vi "device name shot number from tcp udp.vi"(11 "ShotData UDP response":string) -> (1 "all data":string, 2 "shot number":string, 3 "Device name":string)   [LabVIEW 2013]
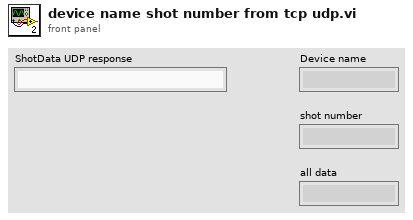
[diagram p1: front panel]
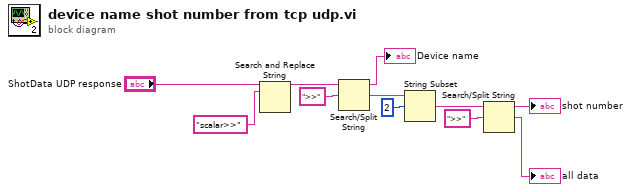
[diagram p0: block diagram]
diagram:
  n1 = Search and Replace String(input string="ShotData UDP response", search string="scalar>>") -> (result string=w3:string)  [unwired: 6 in, 3 out]
  n2 = Search/Split String(string=w3, search string/char (-)=">>") -> (substring before match=→"Device name":string, match + rest of string=w8:string)  [unwired: 1 in, 1 out]
  n3 = String Subset(string=w8, offset (0)=2) -> (substring=w9:string)  [unwired: 1 in]
  n4 = Search/Split String(string=w9, search string/char (-)=">>") -> (substring before match=→"shot number":string, match + rest of string=→"all data":string)  [unwired: 1 in, 1 out]
